vi "Add Port.vi"(7 "Highlight? (F)":bool, 8 "error in":errorcluster, 9 "Port Properties":T1 {"XNET Interface Name" items=["CAN 1", "CAN 2", "CAN 3", "CAN 4", "CAN 5", "CAN 6", "CAN 7", "CAN 8", "CAN 9", "CAN 10", "CAN 11", "CAN 12", "CAN 13", "CAN 14", "CAN 15", "CAN 16"]}, 10 "Port Name":string, 11 "Ports Ref":T3 format="%.0x") -> (0 "error out":errorcluster, 3 "Port Ref out":T3 format="%.0x")   [LabVIEW 2020, in "Communication Bus Template Scripting.lvlib"]
uses:
  Communication Bus Template Scripting.lvlib
  <vilib>/NI VeriStand/Custom Device API/Custom Device Item Ref.ctl
  System Explorer/Implementation/System Explorer/Types/Port Properties.ctl
  System Explorer/Implementation/System Explorer/Types/XNET Interface Name.ctl
  Constants.vi
  <vilib>/NI VeriStand/Custom Device API/Custom Device API.lvlib
  System Explorer/Implementation/Implementation.lvlib
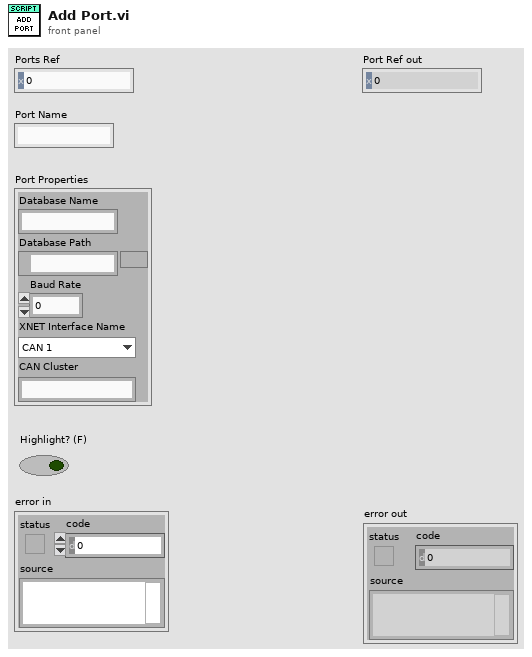
[diagram p1: front panel]
types:
  T1 = typedef "Communication Bus Template System Explorer.lvlib/Implementation.lvlib/Port Properties.ctl" = cluster{"Database Name":string, "Database Path":path, "Baud Rate":u32, "XNET Interface Name":T2, "CAN Cluster":string}
  T2 = typedef "Communication Bus Template System Explorer.lvlib/Implementation.lvlib/XNET Interface Name.ctl" = u16
  T3 = typedef "Custom Device API.lvlib/Custom Device Item Ref.ctl" = u64
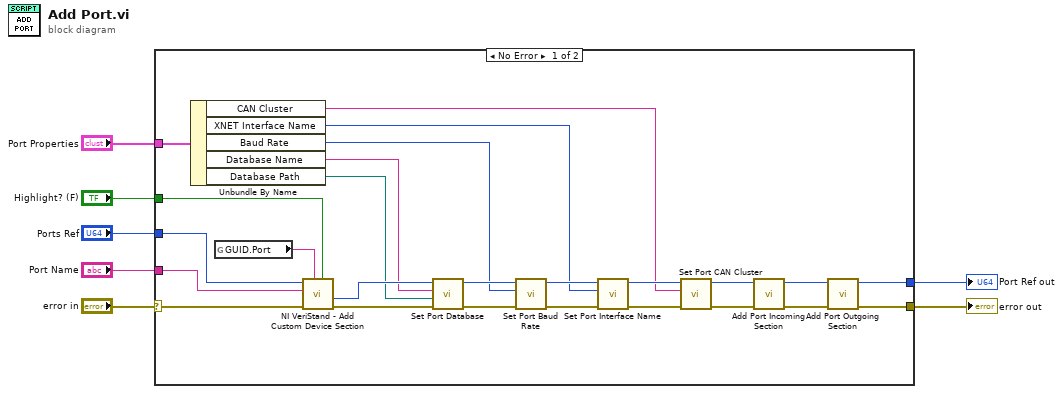
[diagram p0: block diagram]
diagram:
  n1 = case shown="No Error" "error in" {
    selector: "error in" -> [w28 w33]
    tunnel: "Highlight? (F)" -> [w31 _]
    tunnel: "Ports Ref" -> [w30 _]
    tunnel: [w9 w33] -> w5
    tunnel: [w8 _] -> w4
    tunnel: "Port Name" -> [w29 _]
    tunnel: "Port Properties" -> [w23 _]
    frame No Error {
      n2 = Unbundle By Name(w23) -> ("CAN Cluster"=w14:string, "XNET Interface Name"=w15:T2, "Baud Rate"=w20:u32, "Database Name"=w22:string, "Database Path"=w21:path)
      n3 = global read "Constants.vi" "GUID.Port"() -> (w32:string)
      n4 = call <vilib>:"NI VeriStand - Add Custom Device Section.vi"("Highlight? (F)"=w31, "GUID (Default Section)"=w32, "error in (no error)"=w28, "Section Name"=w29, "Parent Ref in"=w30) -> ("error out"=w26:errorcluster, "Section Ptr"=w27:T3)  [unwired: 3 in, 2 out]
      n5 = call "Set Port Database.vi"("error in"=w26, "Database Path"=w21, "Database Name"=w22, "Port Ref"=w27) -> ("error out"=w24:errorcluster, "Port Ref out"=w25:T3)  [unwired: 6 in]
      n6 = call "Set Port Baud Rate.vi"("error in"=w24, "Baud Rate"=w20, "Port Ref"=w25) -> ("error out"=w16:errorcluster, "Port Ref out"=w17:T3)  [unwired: 7 in]
      n7 = call "Set Port Interface Name.vi"("error in"=w16, "XNET Interface Name"=w15, "Port Ref"=w17) -> ("error out"=w19:errorcluster, "Port Ref out"=w18:T3)  [unwired: 7 in]
      n8 = call "Set Port CAN Cluster.vi"("error in"=w19, "CAN Cluster"=w14, "Port Ref"=w18) -> ("error out"=w11:errorcluster, "Port Ref out"=w10:T3)  [unwired: 7 in]
      n9 = call "Add Port Incoming Section.vi"("error in"=w11, "Port Ref"=w10) -> ("error out"=w12:errorcluster, "Port Ref out"=w13:T3)  [unwired: 8 in]
      n10 = call "Add Port Outgoing Section.vi"("error in"=w12, "Port Ref"=w13) -> ("error out"=w9:errorcluster, "Port Ref out"=w8:T3)  [unwired: 8 in]
    }
    frame Error {
    }
  }
  "error out" <- w5
  "Port Ref out" <- w4
